vi "SVI_FH_Parser.vi"(4 "Cluster in":cluster{"Array":dbl[], "Array":dbl[]}, 7 "read buffer":string) -> (0 "Cluster out":cluster{"Array":dbl[], "Array":dbl[]}, 1 "Species":string="Mercury", 2 "Current":dbl, 3 "Scan Voltage (V)":dbl)   [LabVIEW 2014]
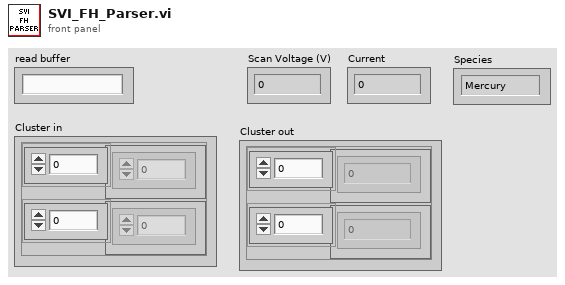
[diagram p1: front panel]
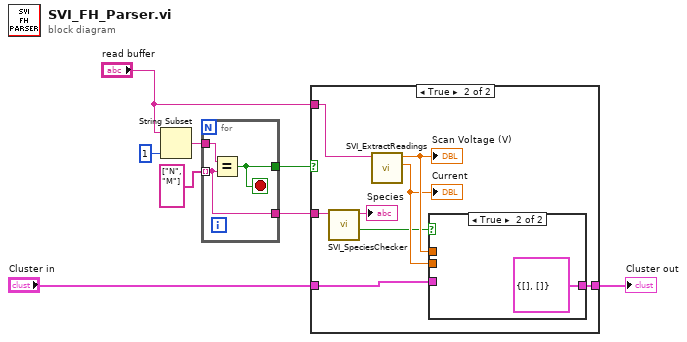
[diagram p0: block diagram]
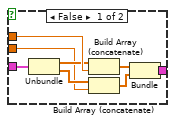
[diagram p3: hidden frame]
diagram:
  n1 = String Subset(string="read buffer", length (rest)=1 ("length (rest)")) -> (substring=w2:string)  [unwired: 1 in]
  n2 = for {
    tunnel: w2 -> [w11]
    tunnel: string[] ["N", "M"] -> [w9] mode=indexing
    tunnel: [w10] -> w4
    tunnel: [w9] -> w5
    stop <- w10 stop-if-true
    n3 = Equal?(x=w11, y=w9) -> (x = y?=w10:bool)
  }
  n4 = case shown="True" w4 {
    tunnel: w5 -> [_ w15]
    tunnel: "read buffer" -> [_ w20]
    tunnel: [w12 w17] -> w7
    tunnel: "Cluster in" -> [w12 w18]
    frame False {
    }
    frame True {
      n5 = call "SVI_SpeciesChecker.vi"("Species in"=w15) -> ("Changed"=w13:bool, "Species out"=→"Species":string)  [unwired: 9 in]
      n6 = call "SVI_ExtractReadings.vi"("read buffer"=w20) -> ("Current"=w16:dbl, "Scan Voltage (V)"=w19:dbl)  [unwired: 9 in]
      "Scan Voltage (V)" <- w19
      "Current" <- w16
      n7 = case shown="True" w13 {
        tunnel: w19 -> [w28 _]
        tunnel: w18 -> [w25 _]
        tunnel: [w22 cluster{dbl[], dbl[]} {[], []}] -> w17
        tunnel: w16 -> [w21 _]
        frame False {
          n8 = Unbundle(w25) -> ("Array"=w24:dbl[], "Array"=w23:dbl[])
          n9 = Build Array (concatenate)(w24, w28) -> (w27:dbl[])
          n10 = Build Array (concatenate)(w23, w21) -> (w26:dbl[])
          n11 = Bundle(w27, w26) -> (w22:cluster{dbl[], dbl[]})  [unwired: 1 in]
        }
        frame True {
        }
      }
    }
  }
  "Cluster out" <- w7
